vi "VentCheck.vi"(8 "error in (no error)":errorcluster, 11 "S2.lvclass":refnum<class "S3.lvclass">) -> (0 "error out":errorcluster)   [LabVIEW 2018, in "S3.lvclass"]
uses:
  S3.lvclass
  S3.lvclass/S3.ctl
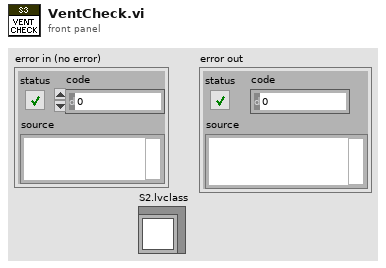
[diagram p1: front panel]
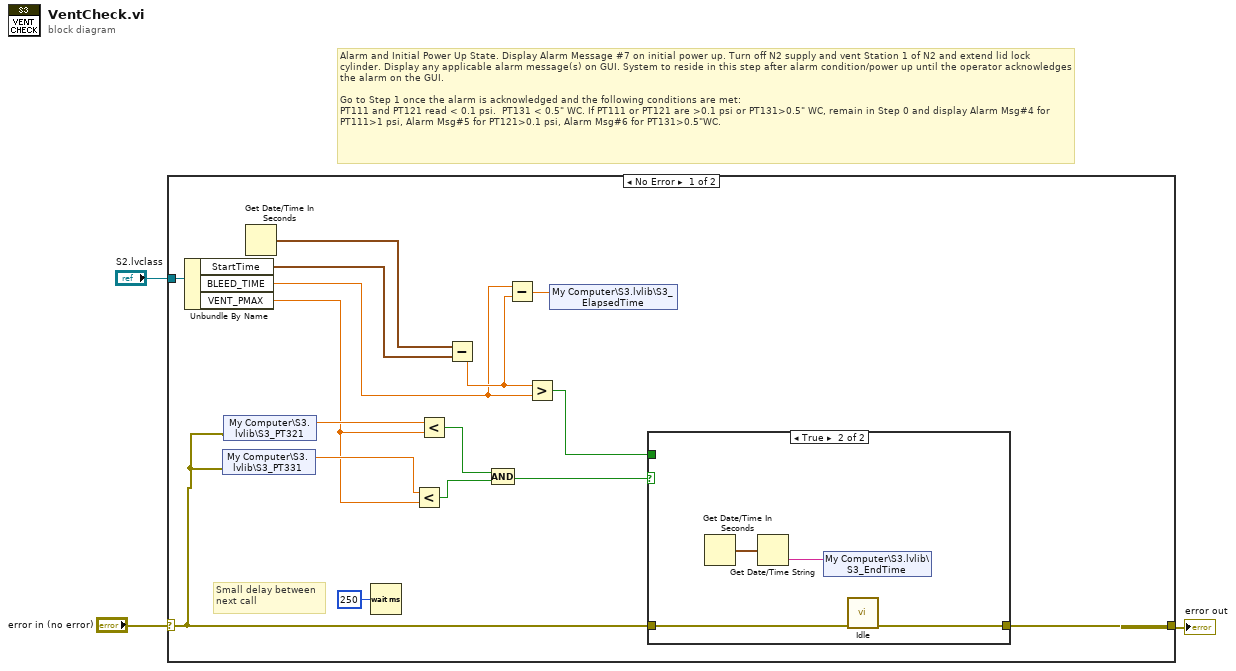
[diagram p0: block diagram]
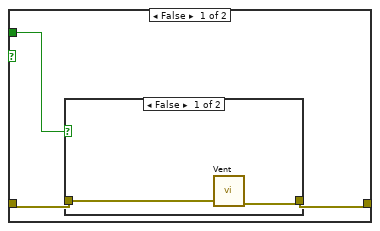
[diagram p2: hidden frame]
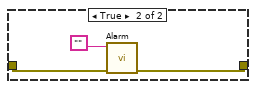
[diagram p3: hidden frame]
diagram:
  # "Alarm and Initial Power Up State. Display Alarm Message #7 on initial power up. Turn off N2 supply and vent Station 1 of N2 and extend lid lock cylinder. Display any applicable alarm message(s) on GUI. System to reside in this step after alarm condition/power up until the operator acknowledges the alarm on the GUI. \n\nGo to Step 1 once the alarm is acknowledged and the following conditions are met:\nPT111 and PT121 read < 0.1 psi.  PT131 < 0.5\" WC. If PT111 or PT121 are >0.1 psi or PT131>0.5\" WC, remain in Step 0 and display Alarm Msg#4 for PT111>1 psi, Alarm Msg#5 for PT121>0.1 psi, Alarm Msg#6 for PT131>0.5\"WC."
  n1 = case shown="No Error" "error in (no error)" {
    selector: "error in (no error)" -> [w7 w32]
    tunnel: [w18 w32] -> w2
    tunnel: "S2.lvclass" -> [w12 _]
    frame No Error {
      # "Small delay between\nnext call"
      n2 = Unbundle By Name(w12) -> ("StartTime"=w11:timestamp, "BLEED_TIME"=w8:dbl, "VENT_PMAX"=w4:dbl)
      n3 = shared-variable "My Computer\\S3.lvlib\\S3_PT331"(error in=w7) -> (w5:dbl)  [unwired: 1 out]
      n4 = shared-variable "My Computer\\S3.lvlib\\S3_PT321"(error in=w7) -> (w6:dbl)  [unwired: 1 out]
      n5 = Get Date/Time In Seconds() -> (seconds since 1Jan1904=w14:timestamp)
      n6 = Wait (ms)(milliseconds to wait=u32 250) -> ()  [unwired: 1 out]
      n7 = Less?(x=w5, y=w4) -> (x < y?=w16:bool)
      n8 = Less?(x=w6, y=w4) -> (x < y?=w17:bool)
      n9 = Subtract(x=w14, y=w11) -> (x-y=w10:dbl)
      n10 = Compound Arithmetic op=AND(w17, w16) -> (w19:bool)
      n11 = Subtract(x=w8, y=w10) -> (x-y=w9:dbl)
      n12 = Greater?(x=w10, y=w8) -> (0:w13:bool)
      n13 = shared-variable "My Computer\\S3.lvlib\\S3_ElapsedTime"(w9) -> ()  [unwired: 1 in, 1 out]
      n14 = case shown="True" w19 {
        tunnel: w7 -> [w21 w31]
        tunnel: [w22 w30] -> w18
        tunnel: w13 -> [w20 _]
        frame False {
          n15 = case shown="False" w20 {
            tunnel: [w23 w27] -> w22
            tunnel: w21 -> [w24 w26]
            frame False {
              n16 = call "Vent.vi"("error in"=w24) -> ("error out"=w23:errorcluster)  [unwired: 10 in]
            }
            frame True {
              n17 = call "Alarm.vi"("error in"=w26, "Alarm"="") -> ("error out"=w27:errorcluster)  [unwired: 9 in]
            }
          }
        }
        frame True {
          n18 = Get Date/Time In Seconds() -> (seconds since 1Jan1904=w29:timestamp)
          n19 = Get Date/Time String(seconds (now)=w29) -> (time string=w28:string)  [unwired: 2 in, 1 out]
          n20 = shared-variable "My Computer\\S3.lvlib\\S3_EndTime"(w28) -> ()  [unwired: 1 in, 1 out]
          n21 = call "Idle.vi"("error in"=w31) -> ("error out"=w30:errorcluster)  [unwired: 10 in]
        }
      }
    }
    frame Error {
    }
  }
  "error out" <- w2
